vi "SetResetRelay.vi"(4 "SetLine":tag="PXI1Slot2/port0/line0", 6 "ResetLine":tag="PXI1Slot2/port0/line1", 8 "milliseconds to wait":u32=10, 11 "Set=T,Rst=F":bool) -> ()   [LabVIEW 2022 SP3]
uses:
  <vilib>/DAQmx/write.llb/DAQmx Write (Digital Bool 1Line 1Point).vi
  <vilib>/DAQmx/create/channels.llb/DAQmx Create Channel (DO-Digital Output).vi
  <vilib>/DAQmx/miscellaneous.llb/DAQmx Fill In Error Info.vi
panel:
  out "Numeric":i32=2
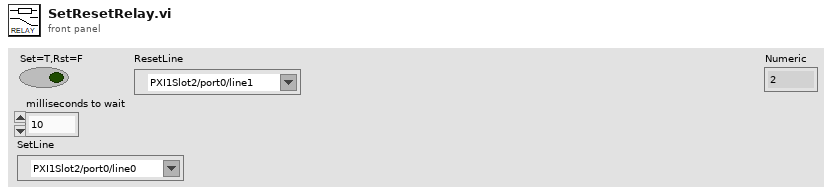
[diagram p1: front panel]
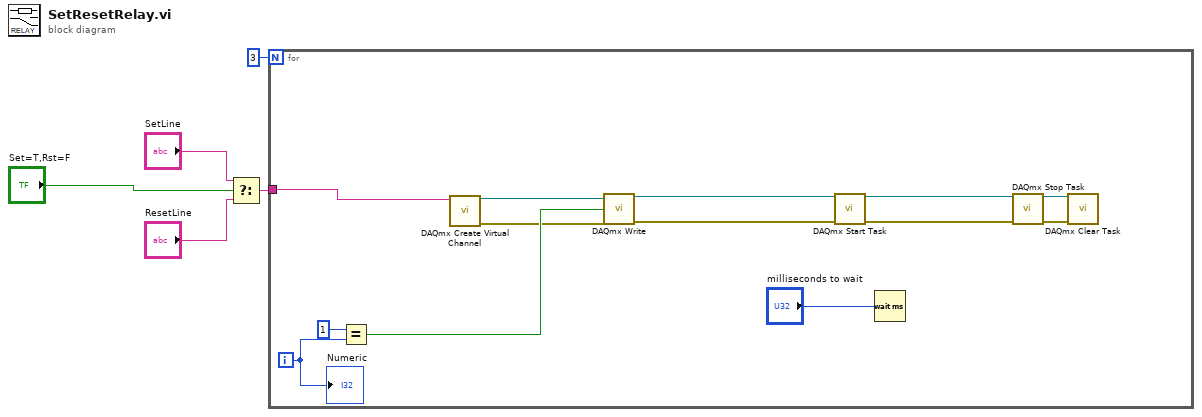
[diagram p0: block diagram]
diagram:
  n1 = Select(t="SetLine", s="Set=T,Rst=F", f="ResetLine") -> (s? t:f=w2:tag)
  n2 = for {
    N: 3 -> [_]
    tunnel: w2 -> [w6]
    i -> [w14]
    n3 = Equal?(x=1, y=w14) -> (x = y?=w12:bool)
    n4 = call-poly <vilib>:"DAQmx Create Virtual Channel.vi"("lines"=w6) -> ("task out"=w18:refnum<k21>, "error out"=w11:errorcluster)  [unwired: 13 in]
    n5 = call-poly <vilib>:"DAQmx Write.vi"("task/channels in"=w18, "data"=w12, "error in"=w11) -> ("task out"=w17:refnum<k21>, "error out"=w10:errorcluster)  [unwired: 10 in, 1 out]
    n6 = call <vilib>:"DAQmx Start Task.vi"("task/channels in"=w17, "error in"=w10) -> ("task out"=w16:refnum<k21>, "error out"=w9:errorcluster)  [unwired: 12 in]
    n7 = Wait (ms)(milliseconds to wait="milliseconds to wait") -> ()  [unwired: 1 out]
    n8 = call <vilib>:"DAQmx Stop Task.vi"("task/channels in"=w16, "error in"=w9) -> ("task out"=w15:refnum<k21>, "error out"=w8:errorcluster)  [unwired: 12 in]
    n9 = call <vilib>:"DAQmx Clear Task.vi"("task in"=w15, "error in"=w8) -> ()  [unwired: 13 in, 1 out]
    "Numeric" <- w14
  }
